vi "create actor FP Queue.vi"(11 "Template in":refnum<class "Template.lvclass">) -> (0 "error out":errorcluster, 3 "Template out":refnum<class "Template.lvclass">)   [LabVIEW 2020, in "Template.lvlib" / "Template.lvclass"]
uses:
  Template.lvclass
  Template.lvclass/Template.ctl
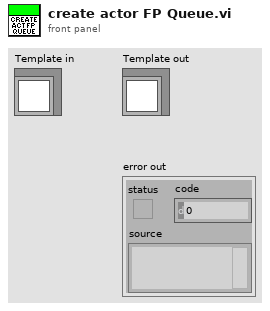
[diagram p1: front panel]
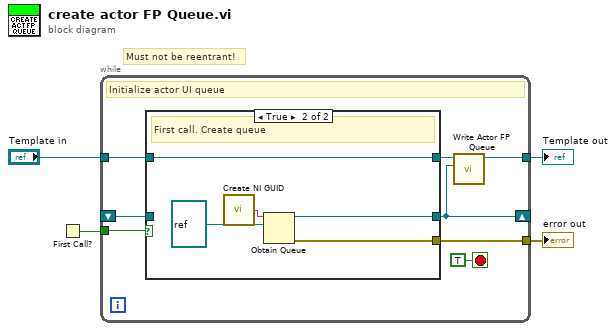
[diagram p0: block diagram]
diagram:
  # "Must not be reentrant!"
  n1 = First Call?() -> (First Call?: T/F=w1:bool)
  n2 = while {
    tunnel: [w11] -> w2
    tunnel: "Template in" -> [w12]
    tunnel: [w7] -> w3
    tunnel: w1 -> [w10]
    shift-right: [w6] -> _
    shift-left: _ -> [w5]
    stop <- TRUE stop-if-true
    # "Initialize actor UI queue"
    n3 = case shown="True" w10 {
      tunnel: w12 -> [w14 w15]
      tunnel: [w14 w15] -> w8
      tunnel: [_ w17] -> w11
      tunnel: [w13 w16] -> w6
      tunnel: w5 -> [w13 _]
      frame False {
        # "Queue has already been created"
      }
      frame True {
        # "First call. Create queue"
        n4 = call <vilib>:"Create NI GUID.vi"() -> ("NI GUID"=w18:string)
        n5 = Obtain Queue(name (unnamed)=w18, element data type=refnum<vi> refnum ("This VI")) -> (queue out=w16:refnum<queue>, error out=w17:errorcluster)  [unwired: 3 in, 1 out]
      }
    }
    n6 = call "Write Actor FP Queue.vi"("Actor FP Queue"=w6, "Template in"=w8) -> ("Template out"=w7:refnum<class "Template.lvclass">)  [unwired: 9 in]
  }
  "error out" <- w2
  "Template out" <- w3
